vi "InternalCoincidenceToSaveCoincidence.vi"(1 "Coincidences":T1[](array[typedef])) -> (0 "Array":T2[](array[typedef]))   [LabVIEW 2016]
uses:
  Typedefs/CoincidenceWithGPSformat.ctl
  Typedefs/Coincidence.ctl
panel:
  out "Boolean":bool
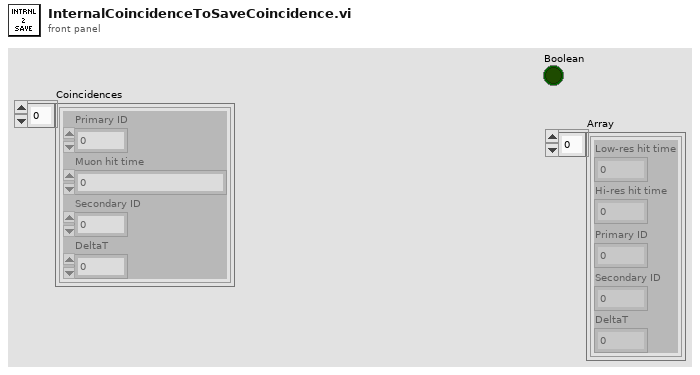
[diagram p1: front panel]
types:
  T1 = typedef "Coincidence.ctl" = cluster{"Primary ID":i8, "Muon hit time":u64, "Secondary ID":i8, "DeltaT":i32}
  T2 = typedef "CoincidenceWithGPSformat.ctl" = cluster{"Low-res hit time":u32, "Hi-res hit time":u32, "Secondary ID":i8, "DeltaT":i32, "Primary ID":i8}
  T3 = enum16{"insertPPS", "insertUTC", "read", "initiate"}
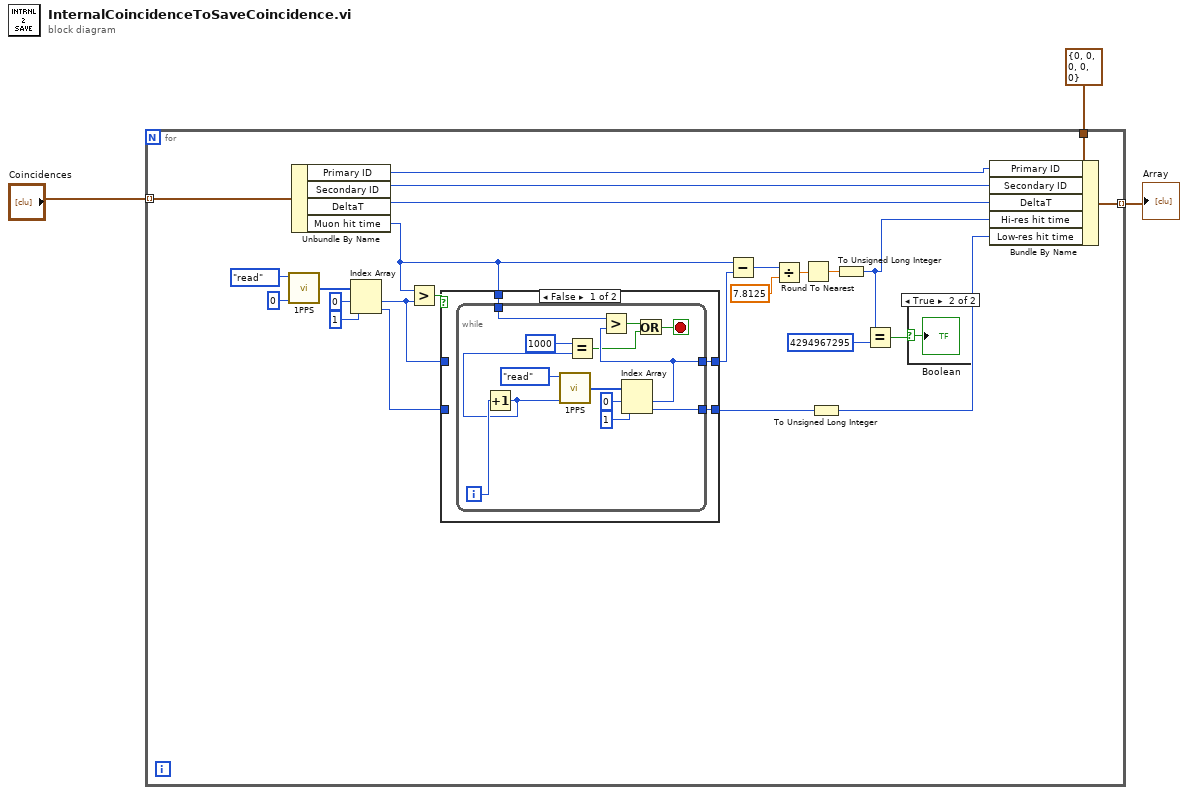
[diagram p0: block diagram]
diagram:
  n1 = for {
    tunnel: "Coincidences" -> [w27] mode=indexing
    tunnel: T2 {"Low-res hit time"=0, "Hi-res hit time"=0, "Secondary ID"=0, "DeltaT"=0, "Primary ID"=0} ("Coincidence") -> [w23]
    tunnel: [w19] -> w1 mode=indexing
    n2 = call "1PPS.vi"("Read Index\nNumber"=0 ("Read Index\nNumber"), "Action"=T3."read") -> ("Array"=w28:u32[])  [unwired: 2 in]
    n3 = Unbundle By Name(w27) -> ("Primary ID"=w14:i8, "Secondary ID"=w22:i8, "DeltaT"=w21:i32, "Muon hit time"=w7:u64)
    n4 = Index Array(array=w28, index #1=0 ("index"), index #2=1 ("index")) -> (element #1=w13:u32, element #2=w10:u32)
    n5 = Greater?(x=w7, y=w13) -> (0:w24:bool)
    n6 = case shown="False" w24 {
      tunnel: [w32 w47] -> w12
      tunnel: w13 -> [_ w47]
      tunnel: w10 -> [_ w46]
      tunnel: [w31 w46] -> w20
      tunnel: w7 -> [w30 _]
      frame False {
        n7 = while {
          tunnel: [w38] -> w32
          tunnel: [w42] -> w31
          tunnel: w30 -> [w39]
          i -> [w40]
          stop <- w33 stop-if-true
          n8 = Increment(x=w40) -> (x+1=w37:i32)
          n9 = call "1PPS.vi"("Read Index\nNumber"=w37, "Action"=T3."read") -> ("Array"=w43:u32[])  [unwired: 2 in]
          n10 = Equal?(x=1000, y=w37) -> (x = y?=w34:bool)
          n11 = Index Array(array=w43, index #1=0 ("index"), index #2=1 ("index")) -> (element #1=w38:u32, element #2=w42:u32)
          n12 = Greater?(x=w39, y=w38) -> (0:w35:bool)
          n13 = Or(x=w35, y=w34) -> (x .or. y?=w33:bool)
        }
      }
      frame True {
      }
    }
    n14 = Subtract(x=w7, y=w12) -> (x-y=w18:u64)
    n15 = Divide(x=w18, y=7.8125) -> (x/y=w16:dbl)
    n16 = Round To Nearest(number=w16) -> (nearest integer value=w15:dbl)
    n17 = To Unsigned Long Integer(number=w20) -> (unsigned 32bit integer=w11:u32)
    n18 = To Unsigned Long Integer(number=w15) -> (unsigned 32bit integer=w6:u32)
    n19 = Equal?(x=w6, y=u32 4294967295) -> (x = y?=w4:bool)
    n20 = case shown="True" w4 {
      selector: w4 -> [_ w29]
      frame False {
      }
      frame True {
        "Boolean" <- w29
      }
    }
    n21 = Bundle By Name(cluster=w23, "Primary ID"=w14, "Secondary ID"=w22, "DeltaT"=w21, "Hi-res hit time"=w6, "Low-res hit time"=w11) -> (w19:T2)
  }
  "Array" <- w1
